vi "Update Offset.vi"(6 "Enabled Site":i32[](array[numeric]), 7 "Calibration Cfg File":T1, 8 "error in":errorcluster, 10 "Final Offset":T3, 11 "CorrOffset File In":T2) -> (0 "error out":errorcluster, 3 "CorrOffset File Out":T2, 5 "Update OK":bool)   [LabVIEW 2020, in "GUCalibration2.lvlib"]
uses:
  GUCalibration2.lvlib
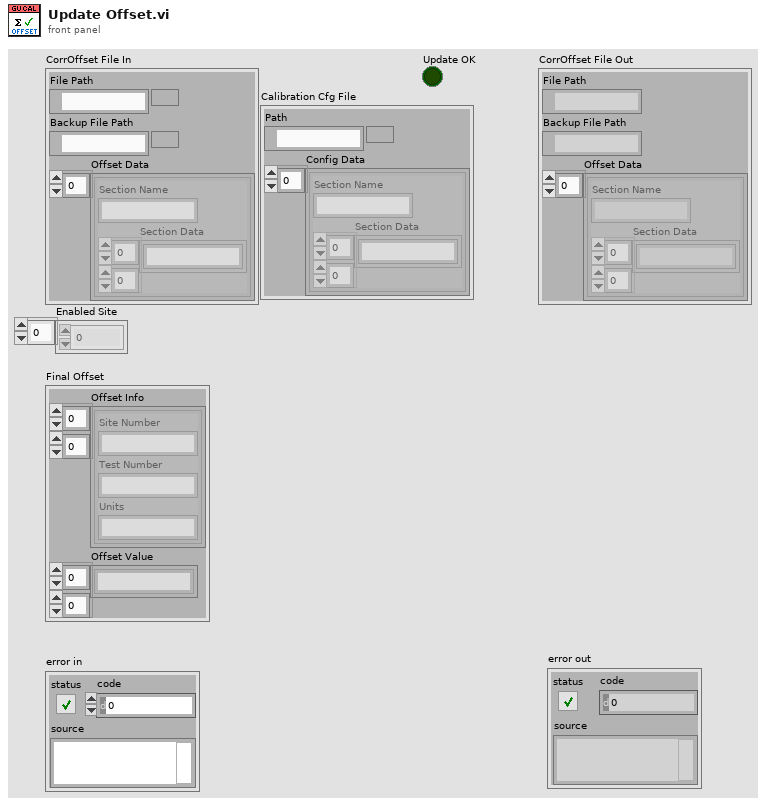
[diagram p1: front panel]
types:
  T1 = cluster{"Path":path, "Config Data":cluster{"Section Name":string, "Section Data":string[][]}[]}
  T2 = cluster{"File Path":path, "Backup File Path":path, "Offset Data":cluster{"Section Name":string, "Section Data":string[][]}[]}
  T3 = cluster{"Offset Info":cluster{"Site Number":string, "Test Number":string, "Units":string}[][], "Offset Value":string[][]}
  T4 = cluster{"Section Name":string, "Section Data":string[][]}[]
  T5 = cluster{"Site Number":string, "Test Number":string, "Units":string}[][]
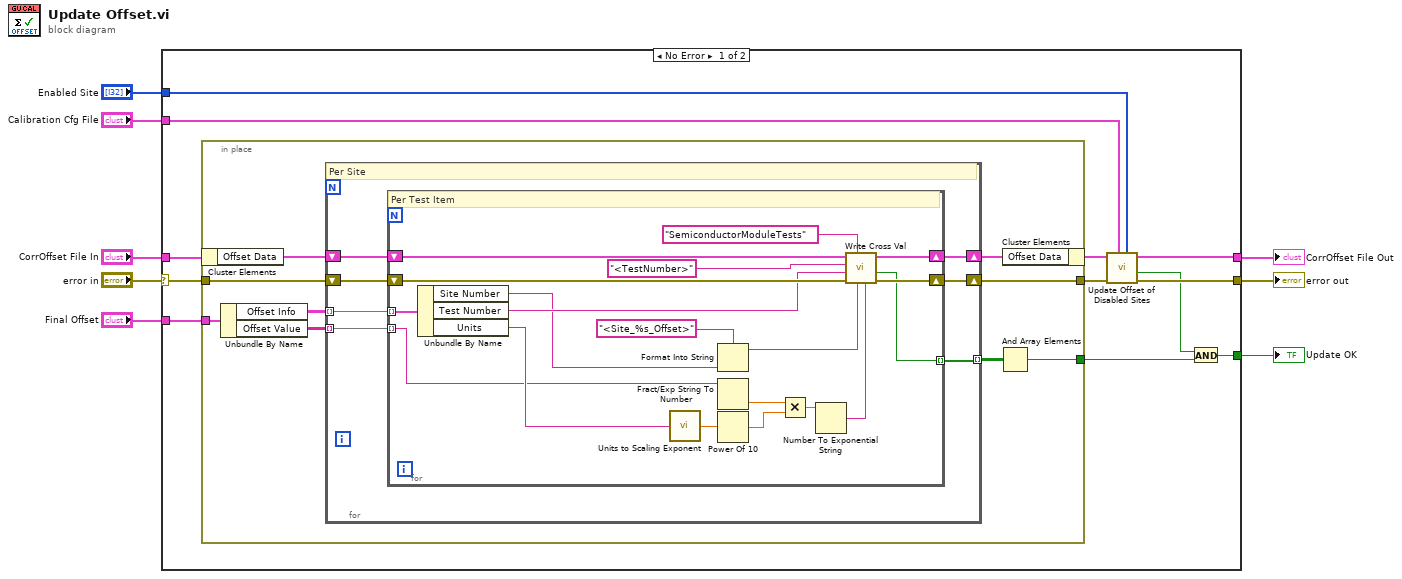
[diagram p0: block diagram]
diagram:
  n1 = case shown="No Error" "error in" {
    selector: "error in" -> [w19 w56]
    tunnel: "CorrOffset File In" -> [w20 w57]
    tunnel: [w13 w57] -> w4
    tunnel: [w16 w56] -> w8
    tunnel: [w10 _] -> w7
    tunnel: "Final Offset" -> [w18 _]
    tunnel: "Calibration Cfg File" -> [w14 _]
    tunnel: "Enabled Site" -> [w9 _]
    frame No Error {
      n2 = in-place {
        in-place-border: w19 -> [w29]
        in-place-border: [w26] -> w17
        in-place-border: [w25] -> w11
        in-place-border: w18 -> [w23]
        n3 = in-place-cluster #1(w20) -> ("Offset Data"=w28:T4)
        n4 = Unbundle By Name(w23) -> ("Offset Info"=w21:T5, "Offset Value"=w22:string[][])
        n5 = for {
          shift-right: [w34] -> w27
          shift-left: w28 -> [w36]
          shift-right: [w33] -> w26
          shift-left: w29 -> [w35]
          tunnel: [w32] -> w24 mode=indexing
          tunnel: w22 -> [w30] mode=indexing
          tunnel: w21 -> [w31] mode=indexing
          # "Per Site"
          n6 = for {
            tunnel: [w48] -> w32 mode=indexing
            shift-right: [w49] -> w33
            shift-left: w35 -> [w54]
            shift-right: [w50] -> w34
            shift-left: w36 -> [w55]
            tunnel: w31 -> [w42] mode=indexing
            tunnel: w30 -> [w39] mode=indexing
            # "Per Test Item"
            n7 = Unbundle By Name(w42) -> ("Site Number"=w37:string, "Test Number"=w40:string, "Units"=w41:string)
            n8 = call "Units to Scaling Exponent.vi"("Units"=w41) -> ("Scaling Exponent"=w47:dbl)  [unwired: 3 in]
            n9 = Format Into String(format string="<Site_%s_Offset>", w37) -> (resulting string=w51:string)  [unwired: 2 in, 1 out]
            n10 = Fract/Exp String To Number(string=w39) -> (number=w45:dbl)  [unwired: 3 in, 1 out]
            n11 = Power Of 10(x=w47) -> (10^x=w46:dbl)
            n12 = Multiply(x=w45, y=w46) -> (x*y=w44:dbl)
            n13 = Number To Exponential String(number=w44) -> (E-format string=w43:string)  [unwired: 3 in]
            n14 = call "Write Cross Val.vi"("Col Header Val 2"=w43, "Col Header Name 2"=w51, "Section Name"="SemiconductorModuleTests", "error in (no error)"=w54, "Col Header Val 1"=w40, "Col Header Name 1"="<TestNumber>", "Config Data"=w55) -> ("error out"=w49:errorcluster, "Find?"=w48:bool, "Config Data dup"=w50:T4)  [unwired: 2 in]
          }
        }
        n15 = And Array Elements(Boolean array=w24) -> (logical AND=w25:bool)
        n16 = in-place-cluster #1("Offset Data"=w27) -> (w15:T2)
      }
      n17 = call "Update Offset of Disabled Sites.vi"("Enabled Sites"=w9, "Calibration Cfg File"=w14, "error in"=w17, "CorrOffset File In"=w15) -> ("error out"=w16:errorcluster, "Update OK"=w12:bool, "CorrOffset File Out"=w13:T2)  [unwired: 5 in]
      n18 = And(x=w12, y=w11) -> (x .and. y?=w10:bool)
    }
    frame Error {
    }
  }
  "error out" <- w8
  "Update OK" <- w7
  "CorrOffset File Out" <- w4
